vi "Write Bool1D A.vi"(8 "error in (no error)":errorcluster, 10 "Abs_Types.lvlib:Boolean.lvclass":refnum<class "Abs_Boolean_1D.lvclass">, 11 "Two Terminal in":refnum<class "AbsFunc_Two Term_Bool_1D.lvclass">) -> (0 "error out":errorcluster, 3 "Two Terminal out":refnum<class "AbsFunc_Two Term_Bool_1D.lvclass">)   [LabVIEW 2021, in "AbsFunc_Two Term_Bool_1D.lvclass"]
uses:
  AbsFunc_Two Term_Bool_1D.lvclass
  Abs_Types/Boolean_1D/Abs_Boolean_1D.lvclass
  AbsFunc_Two Term_Bool_1D.lvclass/AbsFunc_Two Term_Bool_1D.ctl
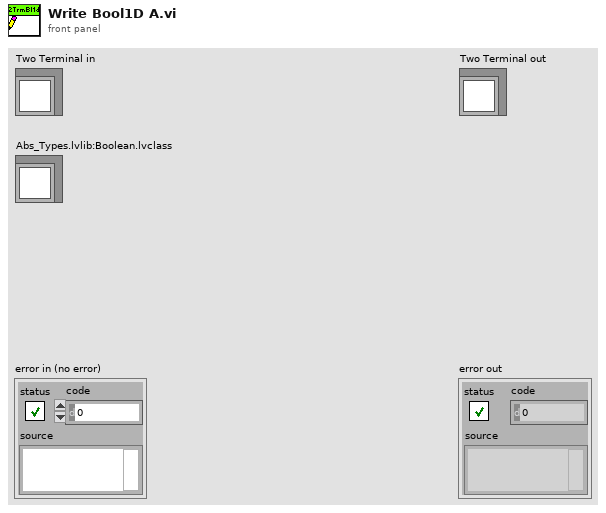
[diagram p1: front panel]
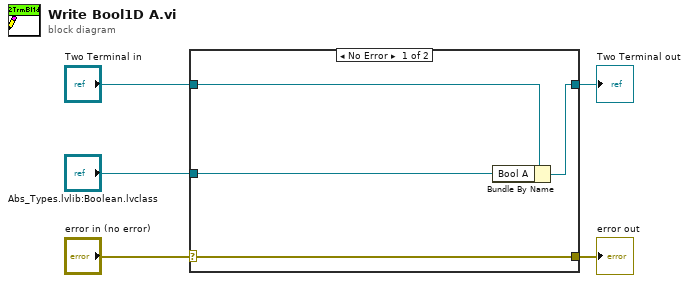
[diagram p0: block diagram]
diagram:
  n1 = case shown="No Error" "error in (no error)" {
    selector: "error in (no error)" -> [w9 w10]
    tunnel: [w9 w10] -> w4
    tunnel: [w7 w11] -> w2
    tunnel: "Two Terminal in" -> [w8 w11]
    tunnel: "Abs_Types.lvlib:Boolean.lvclass" -> [w6 _]
    frame No Error {
      n2 = Bundle By Name(cluster=w8, "Bool A"=w6) -> (w7:refnum<class "AbsFunc_Two Term_Bool_1D.lvclass">)
    }
    frame Error {
    }
  }
  "error out" <- w4
  "Two Terminal out" <- w2
